vi "Memory.Pointer.Numeric.Get power of 2.vi"(8 "error in (no error)":errorcluster, 11 "Memory.Pointer.Numeric in":refnum<class "Memory.Pointer.Numeric.lvclass">) -> (0 "error out":errorcluster, 2 "power of 2":i16, 3 "Memory.Pointer.Numeric out":refnum<class "Memory.Pointer.Numeric.lvclass">)   [LabVIEW 2016, in "LabVIEW Memory Manager.lvlib" / "Memory.Pointer.Numeric.lvclass"]
uses:
  Memory.Pointer.Numeric.lvclass
  Memory.Pointer.Numeric.lvclass/Memory.Pointer.Numeric.ctl
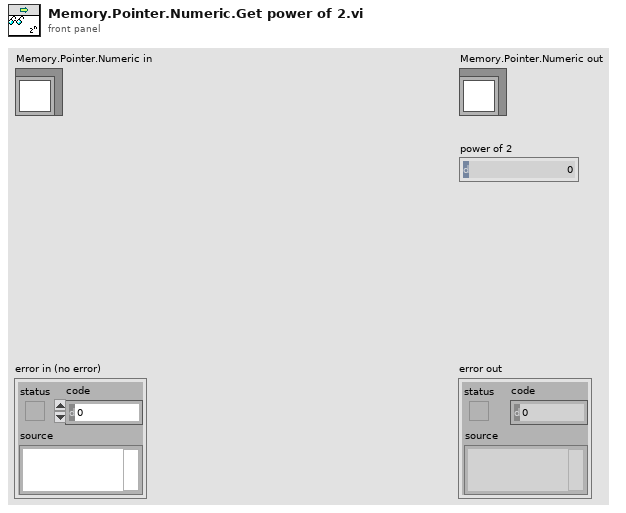
[diagram p1: front panel]
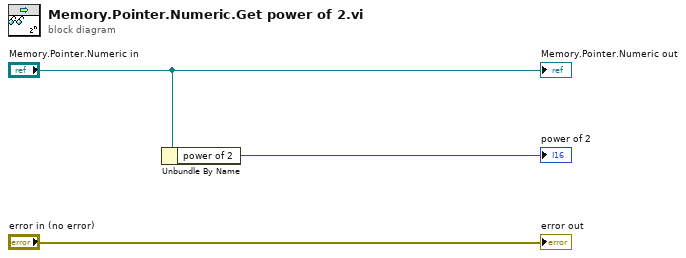
[diagram p0: block diagram]
diagram:
  n1 = Unbundle By Name("Memory.Pointer.Numeric in") -> ("power of 2"=→"power of 2":i16)
  "error out" <- "error in (no error)"
  "Memory.Pointer.Numeric out" <- "Memory.Pointer.Numeric in"
